vi "Connect OPC UA.vi"(8 "error in (no error)":errorcluster, 11 "server endpoint URL":string="opc.tcp://DESKTOP-JA12M0S:49580") -> (0 "error out":errorcluster, 3 "OPC Server Connection":bool)   [LabVIEW 2021]
uses:
  <vilib>/OPCUA/NI OPC UA Client.lvlib
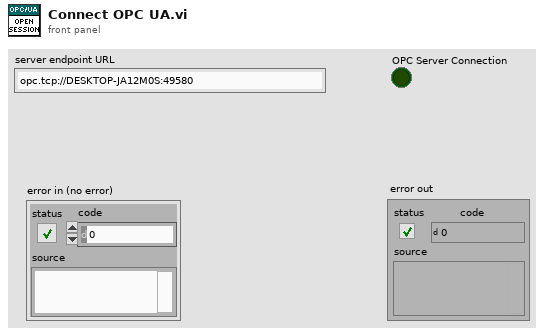
[diagram p1: front panel]
types:
  T1 = typedef "OPC UA Client Refnum.ctl" = refnum<k21>
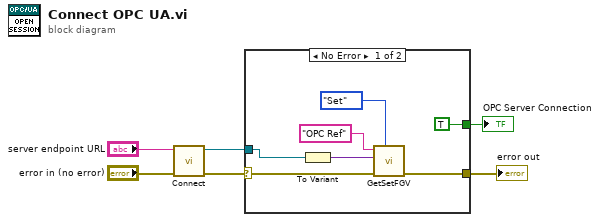
[diagram p0: block diagram]
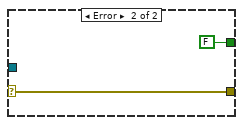
[diagram p2: hidden frame]
diagram:
  n1 = call <vilib>:"Connect.vi"("error in (no error)"="error in (no error)", "server endpoint URL"="server endpoint URL") -> ("error out"=w3:errorcluster, "OPC UA client refnum out"=w4:T1)  [unwired: 7 in, 1 out]
  n2 = case shown="No Error" w3 {
    selector: w3 -> [w11 w15]
    tunnel: [w10 w15] -> w2
    tunnel: w4 -> [w9 _]
    tunnel: [TRUE FALSE] -> w1
    frame No Error {
      n3 = To Variant(anything=w9) -> (Variant=w7:variant)
      n4 = call "GetSetFGV.vi"("Method (Get)"=enum16{"Get", "Set"}."Set", "error in"=w11, "Data In"=w7, "Name"="OPC Ref") -> ("error out"=w10:errorcluster)  [unwired: 6 in, 1 out]
    }
    frame Error {
    }
  }
  "error out" <- w2
  "OPC Server Connection" <- w1
